vi "iniFileDoubleType.vi"(0 "refnum":T1, 1 "default value":dbl, 7 "section":string="RED", 11 "error in (no error)":errorcluster, 12 "key":string) -> (3 "value":dbl, 4 "refnum out":T1, 6 "found?":bool, 8 "section dup":string="RED", 15 "error out":errorcluster)   [LabVIEW 2015]
doc: "Same functionality than LabVIEW Native implementation but this version allows to interconnect same sections between, also default value, key and value in a cleaner way.\n\nDeveloped by Ezequiel Glz. plastilinapps.com"
uses:
  <vilib>/Utility/config.llb/Config Data RefNum.ctl
  <vilib>/Utility/config.llb/Read Key (Double).vi
  <vilib>/Utility/config.llb/NI_LVConfig.lvlib
panel:
  # "Developed by Ezequiel Gonzalez\nPlastilinapps.com 2015"
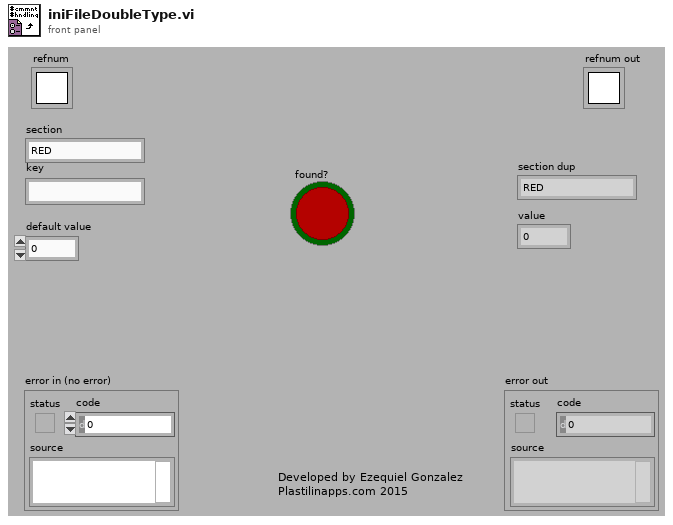
[diagram p1: front panel]
types:
  T1 = typedef "NI_LVConfig.lvlib/Config Data RefNum.ctl" = refnum<k1>
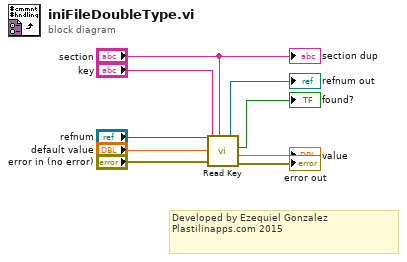
[diagram p0: block diagram]
diagram:
  # "Developed by Ezequiel Gonzalez\nPlastilinapps.com 2015"
  n1 = call-poly <vilib>:"Read Key.vi"("section"="section", "error in (no error)"="error in (no error)", "default value"="default value", "key"="key", "refnum"="refnum") -> ("error out"=→"error out":errorcluster, "value"=→"value":dbl, "found?"=→"found?":bool, "refnum out"=→"refnum out":T1)  [unwired: 3 in]
  "section dup" <- "section"
